vi "Read Sensors.vi"(6 "error in (no error)":errorcluster, 9 "UniCyRO_Host_Sim in":refnum<class "UniCyRO_Host_Sim.lvclass">) -> (0 "error out":errorcluster, 2 "Data":T1, 3 "UniCyRO_Host_Sim out":refnum<class "UniCyRO_Host_Sim.lvclass">)   [LabVIEW 2012, in "UniCyRO.lvlib" / "UniCyRO_Host_Sim.lvclass"]
uses:
  UniCyRO_Host_Sim.lvclass
  UniCyRO_Host_Sim.lvclass/UniCyRO_Host_Sim.ctl
  <instrlib>/Sparkfun Atomic IMU/HAIOL/Sparkfun Atomic IMU.lvclass
  <instrlib>/Hokuyo URG Series/HAIOL/Hokuyo URG Series.lvclass
  <instrlib>/Garmin GPS Series/HAIOL/Garmin GPS Series.lvclass
  <instrlib>/Honeywell Compass HMC6343/HAIOL/Honeywell Compass HMC6343.lvclass
  <vilib>/robotics/Utilities/NI_Robotics Utilities.lvlib
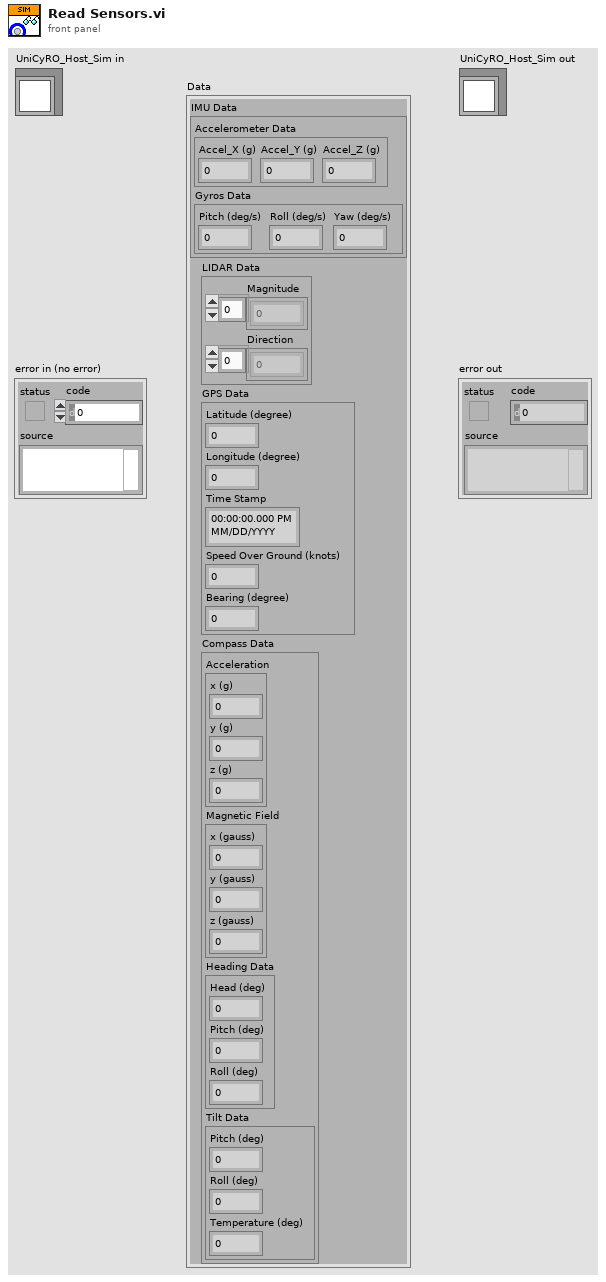
[diagram p1: front panel]
types:
  T1 = cluster{"IMU Data":cluster{"Accelerometer Data":cluster{"Accel_X (g)":dbl, "Accel_Y (g)":dbl, "Accel_Z (g)":dbl}, "Gyros Data":cluster{"Pitch (deg/s)":dbl, "Roll (deg/s)":dbl, "Yaw (deg/s)":dbl}}, "LIDAR Data":cluster{"Magnitude":dbl[], "Direction":dbl[]}, "GPS Data":cluster{"Latitude (degree)":dbl, "Longitude (degree)":dbl, "Time Stamp":timestamp, "Speed Over Ground (knots)":dbl, "Bearing (degree)":dbl}, "Compass Data":cluster{"Acceleration":cluster{"x (g)":dbl, "y (g)":dbl, "z (g)":dbl}, "Magnetic Field":cluster{"x (gauss)":dbl, "y (gauss)":dbl, "z (gauss)":dbl}, "Heading Data":cluster{"Head (deg)":dbl, "Pitch (deg)":dbl, "Roll (deg)":dbl}, "Tilt Data":cluster{"Pitch (deg)":dbl, "Roll (deg)":dbl, "Temperature (deg)":dbl}}}
  T2 = cluster{"Acceleration":cluster{"x (g)":dbl, "y (g)":dbl, "z (g)":dbl}, "Magnetic Field":cluster{"x (gauss)":dbl, "y (gauss)":dbl, "z (gauss)":dbl}, "Heading Data":cluster{"Head (deg)":dbl, "Pitch (deg)":dbl, "Roll (deg)":dbl}, "Tilt Data":cluster{"Pitch (deg)":dbl, "Roll (deg)":dbl, "Temperature (deg)":dbl}}
  T3 = cluster{"Latitude (degree)":dbl, "Longitude (degree)":dbl, "Time Stamp":timestamp, "Speed Over Ground (knots)":dbl, "Bearing (degree)":dbl}
  T4 = cluster{"Accelerometer Data":cluster{"Accel_X (g)":dbl, "Accel_Y (g)":dbl, "Accel_Z (g)":dbl}, "Gyros Data":cluster{"Pitch (deg/s)":dbl, "Roll (deg/s)":dbl, "Yaw (deg/s)":dbl}}
  T5 = cluster{"Pitch (deg/s)":dbl, "Roll (deg/s)":dbl, "Yaw (deg/s)":dbl}
  T6 = cluster{"Accel_X (g)":dbl, "Accel_Y (g)":dbl, "Accel_Z (g)":dbl}
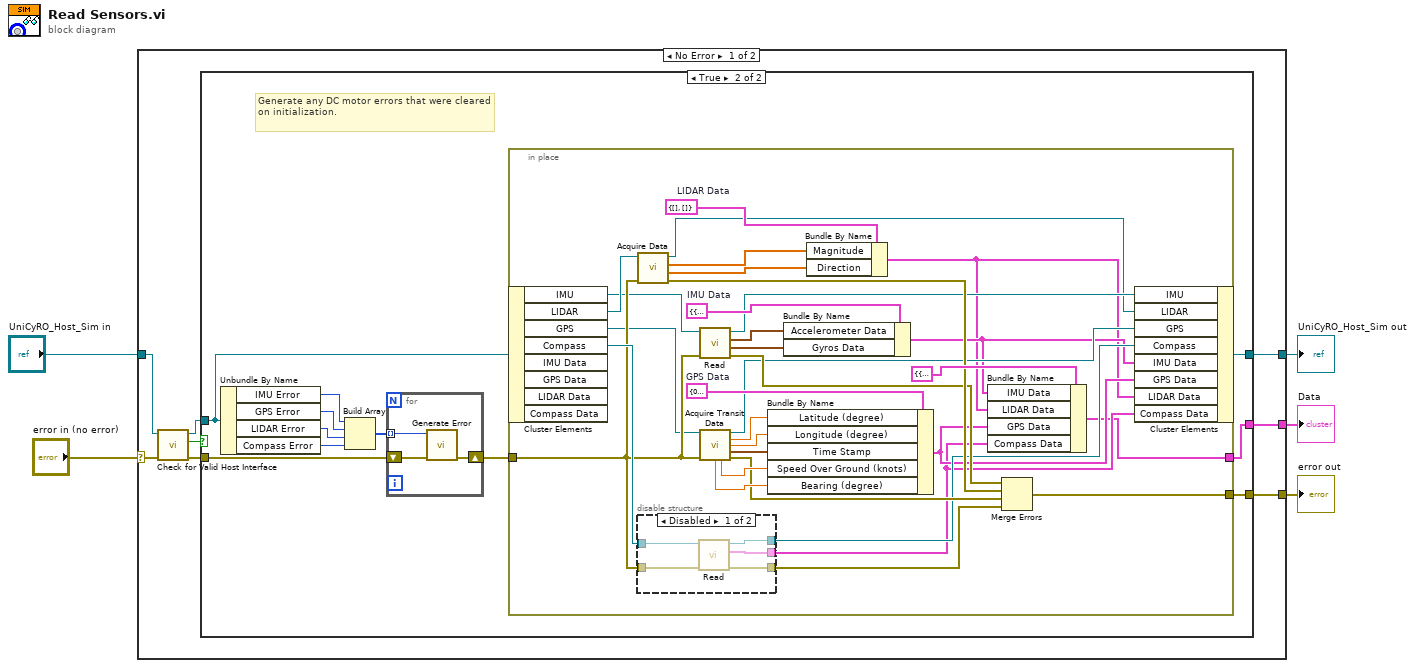
[diagram p0: block diagram]
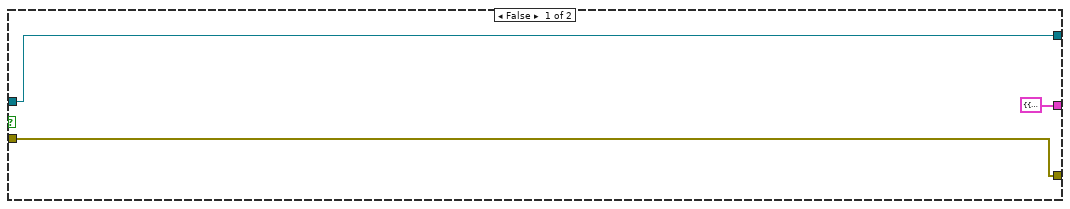
[diagram p2: hidden frame]
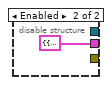
[diagram p3: hidden frame]
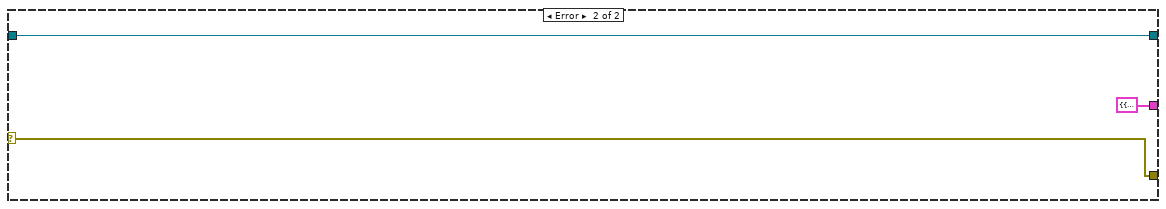
[diagram p4: hidden frame]
diagram:
  n1 = case shown="No Error" "error in (no error)" {
    selector: "error in (no error)" -> [w10 w71]
    tunnel: [w12 w71] -> w2
    tunnel: [w13 w70] -> w4
    tunnel: "UniCyRO_Host_Sim in" -> [w6 w70]
    tunnel: [w7 T1 {"IMU Data"={"Accelerometer Data"={"Accel_X (g)"=0.0, "Accel_Y (g)"=0.0, "Accel_Z (g)"=0.0}, "Gyros Data"={"Pitch (deg/s)"=0.0, "Roll (deg/s)"=0.0, "Yaw (deg/s)"=0.0}}, "LIDAR Data"={"Magnitude"=[], "Direction"=[]}, "GPS Data"={"Latitude (degree)"=0.0, "Longitude (degree)"=0.0, "Time Stamp"=timestamp(0 s since 1904-01-01), "Speed Over Ground (knots)"=0.0, "Bearing (degree)"=0.0}, "Compass Data"={"Acceleration"={"x (g)"=0.0, "y (g)"=0.0, "z (g)"=0.0}, "Magnetic Field"={"x (gauss)"=0.0, "y (gauss)"=0.0, "z (gauss)"=0.0}, "Heading Data"={"Head (deg)"=0.0, "Pitch (deg)"=0.0, "Roll (deg)"=0.0}, "Tilt Data"={"Pitch (deg)"=0.0, "Roll (deg)"=0.0, "Temperature (deg)"=0.0}}} ("Data")] -> w1
    frame No Error {
      n2 = call "Check for Valid Host Interface.vi"("error in (no error)"=w10, "UniCyRO_Host_Sim in"=w6) -> ("error out"=w9:errorcluster, "valid?"=w8:bool, "UniCyRO_Host_Sim out"=w11:refnum<class "UniCyRO_Host_Sim.lvclass">)  [unwired: 7 in]
      n3 = case shown="True" w8 {
        tunnel: [w16 w20] -> w13
        tunnel: [w15 w19] -> w12
        tunnel: w9 -> [w15 w23]
        tunnel: w11 -> [w16 w17]
        tunnel: [T1 {"IMU Data"={"Accelerometer Data"={"Accel_X (g)"=0.0, "Accel_Y (g)"=0.0, "Accel_Z (g)"=0.0}, "Gyros Data"={"Pitch (deg/s)"=0.0, "Roll (deg/s)"=0.0, "Yaw (deg/s)"=0.0}}, "LIDAR Data"={"Magnitude"=[], "Direction"=[]}, "GPS Data"={"Latitude (degree)"=0.0, "Longitude (degree)"=0.0, "Time Stamp"=timestamp(0 s since 1904-01-01), "Speed Over Ground (knots)"=0.0, "Bearing (degree)"=0.0}, "Compass Data"={"Acceleration"={"x (g)"=0.0, "y (g)"=0.0, "z (g)"=0.0}, "Magnetic Field"={"x (gauss)"=0.0, "y (gauss)"=0.0, "z (gauss)"=0.0}, "Heading Data"={"Head (deg)"=0.0, "Pitch (deg)"=0.0, "Roll (deg)"=0.0}, "Tilt Data"={"Pitch (deg)"=0.0, "Roll (deg)"=0.0, "Temperature (deg)"=0.0}}} ("Data") w18] -> w7
        frame False {
        }
        frame True {
          # "Generate any DC motor errors that were cleared on initialization."
          n4 = Unbundle By Name(w17) -> ("IMU Error"=w26:i32, "GPS Error"=w25:i32, "LIDAR Error"=w24:i32, "Compass Error"=w22:i32)
          n5 = Build Array(w26, w25, w24, w22) -> (w27:i32[])
          n6 = for {
            shift-right: [w67] -> w21
            shift-left: w23 -> [w68]
            tunnel: w27 -> [w66] mode=indexing
            n7 = call <vilib>:"Generate Error.vi"("error in (no error)"=w68, "code"=w66) -> ("error out"=w67:errorcluster)  [unwired: 9 in]
          }
          n8 = in-place {
            in-place-border: w21 -> [w41]
            in-place-border: [w40] -> w19
            in-place-border: [w31] -> w18
            w52 = T3 {"Latitude (degree)"=0.0, "Longitude (degree)"=0.0, "Time Stamp"=timestamp(0 s since 1904-01-01), "Speed Over Ground (knots)"=0.0, "Bearing (degree)"=0.0}  # GPS Data
            w49 = cluster{"Magnitude":dbl[], "Direction":dbl[]} {"Magnitude"=[], "Direction"=[]}  # LIDAR Data
            w46 = T4 {"Accelerometer Data"={"Accel_X (g)"=0.0, "Accel_Y (g)"=0.0, "Accel_Z (g)"=0.0}, "Gyros Data"={"Pitch (deg/s)"=0.0, "Roll (deg/s)"=0.0, "Yaw (deg/s)"=0.0}}  # IMU Data
            n9 = in-place-cluster #1(w17) -> ("IMU"=w28:refnum<class "Sparkfun Atomic IMU.lvclass">, "LIDAR"=w30:refnum<class "Hokuyo URG Series.lvclass">, "GPS"=w29:refnum<class "Garmin GPS Series.lvclass">, "Compass"=w42:refnum<class "Honeywell Compass HMC6343.lvclass">)  [unwired: 4 out]
            n10 = call-dynamic "Acquire Data.vi"("error in (no error)"=w41, "Hokuyo URG Series in"=w30) -> ("error out"=w44:errorcluster, "Direction"=w51:dbl[], "Magnitude"=w50:dbl[], "Hokuyo URG Series out"=w38:refnum<class "Hokuyo URG Series.lvclass">)  [unwired: 6 in]
            n11 = disable-structure shown="Disabled" {
              disable-tunnel: w42 -> [w64 _]
              disable-tunnel: [w63 _] -> w36
              disable-tunnel: w41 -> [w62 _]
              disable-tunnel: [w61 _] -> w59
              disable-tunnel: [w60 T2 {"Acceleration"={"x (g)"=0.0, "y (g)"=0.0, "z (g)"=0.0}, "Magnetic Field"={"x (gauss)"=0.0, "y (gauss)"=0.0, "z (gauss)"=0.0}, "Heading Data"={"Head (deg)"=0.0, "Pitch (deg)"=0.0, "Roll (deg)"=0.0}, "Tilt Data"={"Pitch (deg)"=0.0, "Roll (deg)"=0.0, "Temperature (deg)"=0.0}} ("Data")] -> w32
              frame Disabled {
                n12 = call <instrlib>:"Read.vi"("error in (no error)"=w62, "Honeywell Compass HMC6343"=w64) -> ("error out"=w61:errorcluster, "Data"=w60:T2, "Honeywell Compass HMC6343 out"=w63:refnum<class "Honeywell Compass HMC6343.lvclass">)  [unwired: 7 in]
              }
              frame Enabled {
              }
            }
            n13 = call-dynamic <instrlib>:"Read.vi"("error in (no error)"=w41, "Sparkfun Atomic IMU in"=w28) -> ("error out"=w43:errorcluster, "Gyros Data"=w48:T5, "Accelerometer Data"=w47:T6, "Sparkfun Atomic IMU out"=w39:refnum<class "Sparkfun Atomic IMU.lvclass">)  [unwired: 6 in]
            n14 = call-dynamic "Acquire Transit Data.vi"("Garmin GPS Series In"=w29, "error in (no error)"=w41) -> ("Garmin GPS Series Out"=w37:refnum<class "Garmin GPS Series.lvclass">, "Latitude (degree)"=w53:dbl, "Longitude (degree)"=w54:dbl, "Time Stamp"=w55:timestamp, "Bearing (degree)"=w57:dbl, "Speed Over Ground (knots)"=w56:dbl, "error out"=w45:errorcluster)  [unwired: 7 in]
            n15 = Bundle By Name(cluster=w52, "Latitude (degree)"=w53, "Longitude (degree)"=w54, "Time Stamp"=w55, "Speed Over Ground (knots)"=w56, "Bearing (degree)"=w57) -> (w34:T3)
            n16 = Bundle By Name(cluster=w46, "Accelerometer Data"=w47, "Gyros Data"=w48) -> (w35:T4)
            n17 = Bundle By Name(cluster=w49, "Magnitude"=w50, "Direction"=w51) -> (w33:cluster{"Magnitude":dbl[], "Direction":dbl[]})
            n18 = Bundle By Name(cluster=T1 {"IMU Data"={"Accelerometer Data"={"Accel_X (g)"=0.0, "Accel_Y (g)"=0.0, "Accel_Z (g)"=0.0}, "Gyros Data"={"Pitch (deg/s)"=0.0, "Roll (deg/s)"=0.0, "Yaw (deg/s)"=0.0}}, "LIDAR Data"={"Magnitude"=[], "Direction"=[]}, "GPS Data"={"Latitude (degree)"=0.0, "Longitude (degree)"=0.0, "Time Stamp"=timestamp(0 s since 1904-01-01), "Speed Over Ground (knots)"=0.0, "Bearing (degree)"=0.0}, "Compass Data"={"Acceleration"={"x (g)"=0.0, "y (g)"=0.0, "z (g)"=0.0}, "Magnetic Field"={"x (gauss)"=0.0, "y (gauss)"=0.0, "z (gauss)"=0.0}, "Heading Data"={"Head (deg)"=0.0, "Pitch (deg)"=0.0, "Roll (deg)"=0.0}, "Tilt Data"={"Pitch (deg)"=0.0, "Roll (deg)"=0.0, "Temperature (deg)"=0.0}}} ("Data"), "IMU Data"=w35, "LIDAR Data"=w33, "GPS Data"=w34, "Compass Data"=w32) -> (w31:T1)
            n19 = Merge Errors(w43, w44, w45, w59) -> (w40:errorcluster)
            n20 = in-place-cluster #1("IMU"=w39, "LIDAR"=w38, "GPS"=w37, "Compass"=w36, "IMU Data"=w35, "GPS Data"=w34, "LIDAR Data"=w33, "Compass Data"=w32) -> (w20:refnum<class "UniCyRO_Host_Sim.lvclass">)
          }
        }
      }
    }
    frame Error {
    }
  }
  "error out" <- w2
  "UniCyRO_Host_Sim out" <- w4
  "Data" <- w1
